vi "Immediate Measure Single.vi"(8 "error in (no error)":errorcluster, 9 "Max Time (-1ms)":i32=-1, 11 "NI DMM Driver in":refnum<class "DMM.NI.lvclass">) -> (0 "error dub":errorcluster, 1 "Valid measurement?":bool, 2 "Measurement":dbl=nan, 3 "NI DMM Driver out":refnum<class "DMM.NI.lvclass">, 5 "Finished?":bool)   [LabVIEW 2020, in "NI DMM Driver.lvlib" / "DMM.NI.lvclass"]
doc: "Perform a single measurement on the DMM. \nIf the measurement does not complete due to a timeout 'Finished' is set to FALSE, this should not result in an error!\nIf the measurement is valid 'Valid measurement' is set to TRUE."
uses:
  DMM.NI.lvclass
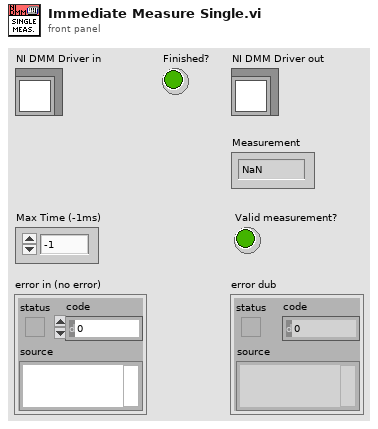
[diagram p1: front panel]
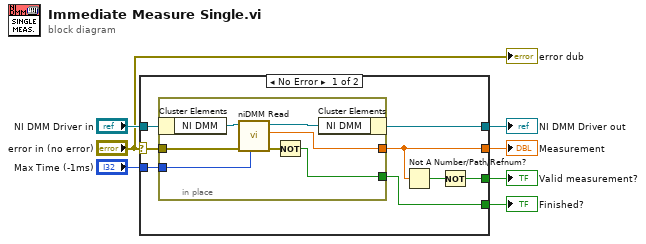
[diagram p0: block diagram]
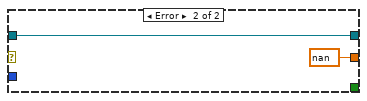
[diagram p2: hidden frame]
diagram:
  n1 = case shown="No Error" "error in (no error)" {
    selector: "error in (no error)" -> [w13 _]
    tunnel: [w14 w24] -> w6
    tunnel: "NI DMM Driver in" -> [w15 w24]
    tunnel: "Max Time (-1ms)" -> [w12 _]
    tunnel: [w10 _] -> w4
    tunnel: [w9 _] -> w3
    tunnel: [w8 nan ("Measurement")] -> w1
    frame No Error {
      n2 = in-place {
        in-place-border: w13 -> [w18]
        in-place-border: w12 -> [w20]
        in-place-border: [w19] -> w8
        in-place-border: [w16] -> w9
        n3 = in-place-cluster #1(w15) -> ("NI DMM"=w22:refnum<k15>)
        n4 = call <instrlib>:"niDMM Read.vi"("Maximum Time (msec)"=w20, "error in (no error)"=w18, "instrument handle"=w22) -> ("error out"=w17:errorcluster, "Measurement"=w19:dbl, "instrument handle out"=w21:refnum<k15>)  [unwired: 6 in]
        n5 = Not(x=w17) -> (.not. x?=w16:bool)
        n6 = in-place-cluster #1("NI DMM"=w21) -> (w14:refnum<class "DMM.NI.lvclass">)
      }
      n7 = Not A Number/Path/Refnum?(number/path/refnum=w8) -> (NaN/Path/Refnum?=w11:bool)
      n8 = Not(x=w11) -> (.not. x?=w10:bool)
    }
    frame Error {
    }
  }
  "NI DMM Driver out" <- w6
  "Measurement" <- w1
  "Valid measurement?" <- w4
  "Finished?" <- w3
  "error dub" <- "error in (no error)"
